vi "Teleop.vi"(10 "Match Info":T2={"Autonomous Elapsed Seconds"=0.0, "TeleOp Elapsed Seconds"=0.0, "Disabled Elapsed Seconds"=0.0, "Visited Autonomous"=FALSE, "Visited TeleOp"=FALSE, "Visited Disabled"=FALSE, "Autonomous Settings"={"Autonomous Style"=enum."Independent", "VI Refnum"=refnum}}, 11 "Call Context":T3) -> ()   [LabVIEW 2020]
doc: "This VI is called for each TeleOp packet received from the DS where the robot is not disabled. It is often used to read from the joysticks and update I/O or to update setpoints for timed control loops. It should complete and return within 20 milliseconds or it may miss DS packets."
uses:
  <vilib>/Rock Robotics/Network Tables/NT Write Numeric Array.vi
  <vilib>/Rock Robotics/Network Tables/NT Write Boolean Array.vi
  <vilib>/Rock Robotics/Network Tables/NT Read Boolean.vi
  <vilib>/Rock Robotics/WPI/ThirdParty/Phoenix-LabVIEW/Motor Controller/Controls/CTRE_Phoenix_MotorControl_ControlMode.ctl
  <vilib>/Rock Robotics/WPI/RobotDrive/WPI_RobotDriveMecanumDrive_Cartesian.vi
  <vilib>/Rock Robotics/Network Tables/NT Read Number.vi
  <vilib>/Rock Robotics/WPI/Solenoid/WPI_SolenoidSetEnum.vi
  <vilib>/Rock Robotics/WPI/DriverStation/WPI_DriverStationMatch Info.ctl
  <vilib>/Rock Robotics/WPI/DriverStation/WPI_DriverStationDerivedRobotMode.ctl
  <vilib>/Rock Robotics/WPI/Solenoid/WPI_SolenoidValue.ctl
panel:
  out "Distance 2":dbl
  out "Distance":dbl
  out "Angle":dbl=360.0
  in  "Camera servo up":i32
  out "Index Reverse":bool
  out "Index Foward":bool
  in  "Indexer Reverse":i32=6
  in  "Indexer forward":i32=4
  out "climb_cylinder":T1
  out "intake_cylinder":T1
  out "Indexer":dbl
  out "intake_motor_output":dbl
  out "Sample Slider 0":dbl(slide) scale=0.0..5.0
  out "Sample Boolean 1":bool
  out "Sample Boolean 0":bool
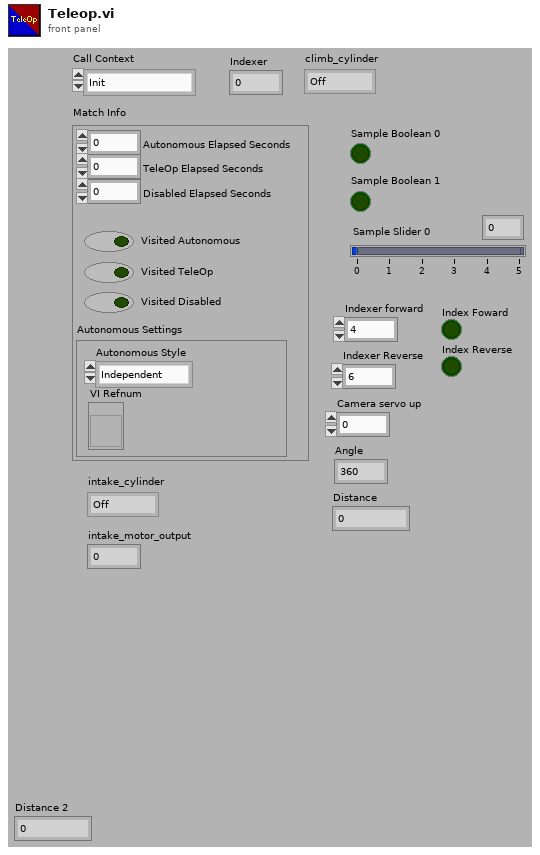
[diagram p1: front panel]
types:
  T1 = typedef "WPI_SolenoidValue.ctl" = enum16{"Off", "On", "Forward", "Reverse"}
  T2 = typedef "WPI_DriverStationMatch Info.ctl" = cluster{"Autonomous Elapsed Seconds":dbl, "TeleOp Elapsed Seconds":dbl, "Disabled Elapsed Seconds":dbl, "Visited Autonomous":bool, "Visited TeleOp":bool, "Visited Disabled":bool, "Autonomous Settings":cluster{"Autonomous Style":enum16{"Iterative", "Independent"}, "VI Refnum":refnum<vi>}}
  T3 = typedef "WPI_DriverStationDerivedRobotMode.ctl" = enum16{"Init", "Execute", "Stop"}
  T4 = typedef "CTRE_Phoenix_MotorControl_ControlMode.ctl" = u16
  T5 = typedef "WPI_GyroDevRef.ctl" = cluster{"DevStatus":errorcluster, "Analog Channel":T6, "Gain (VoltsPerDegree/Second)":dbl, "Gyro Type":enum16{"Analog", "XRS450"}, "Handle":i32, "SPI Bus":T7, "Device Found":bool, "Sample Rate":dbl, "Calibrate On Open":bool, "Offset":dbl}
  T6 = typedef "FPGA_AIChannel.ctl" = enum8{"AI 0", "AI 1", "AI 2", "AI 3", "AI MXP 0", "AI MXP 1", "AI MXP 2", "AI MXP 3", "Invalid"}
  T7 = typedef "spi_bus.ctl" = enum16{"SPI On-Board, CS0", "SPI On-Board, CS1", "SPI On-Board, CS2", "SPI On-Board, CS3", "SPI MXP", "Invalid"}
  T8 = typedef "WPI_EncoderDevRef.ctl" = cluster{"DevStatus":errorcluster, "EncoderIndex":T9, "CounterIndex":T10, "DistancePerCount":dbl, "Decoding Type":T11}
  T9 = typedef "FPGA_EncoderIdx.ctl" = enum8{"Enc 0", "Enc 1", "Enc 2", "Enc 3", "Enc 4", "Enc 5", "Enc 6", "Enc 7", "Invalid"}
  T10 = typedef "FPGA_CounterCtrSystemIndex.ctl" = enum8{"Ctr 0", "Ctr 1", "Ctr 2", "Ctr 3", "Ctr 4", "Ctr 5", "Ctr 6", "Ctr 7", "Invalid"}
  T11 = typedef "WPI_EncoderType.ctl" = enum16{"1x", "2x", "4x"}
  T12 = typedef "WPI_RobotDriveDevRef.ctl" = cluster{"DevStatus":errorcluster, "Motors[]":T13[], "Square Inputs":bool, "Max Output":dbl}
  T13 = typedef "WPI_MotorControlDeviceRef.ctl" = cluster{"DeviceStatus":errorcluster, "Type":T14, "PWM":cluster{"PWM Channel":T15, "DeadBand":T16}, "CAN":cluster{"Device Number":u8, "SetOutput VI Ref":variant, "GetOutput VI Ref":variant, "Enable VI Ref":variant, "Disable VI Ref":variant, "Data":variant}, "Invert":bool, "DIO PWM":cluster{"PWM \"Enable\" Channel":T15, "DIOChannel":T17, "PWM Rate":dbl}}
  T14 = typedef "WPI_MotorControlType.ctl" = enum16{"PWM", "CAN", "DIO PWM"}
  T15 = typedef "FPGA_DIOPWMChannel.ctl" = enum8{"PWM 0", "PWM 1", "PWM 2", "PWM 3", "PWM 4", "PWM 5", "PWM 6", "PWM 7", "PWM 8", "PWM 9", "PWM MXP 0", "PWM MXP 1", "PWM MXP 2", "PWM MXP 3", "PWM MXP 4", "PWM MXP 5", "PWM MXP 6", "PWM MXP 7", "PWM MXP 8", "PWM MXP 9", "Invalid"}
  T16 = typedef "WPI_PWMDeadband.ctl" = cluster{"Name":string, "maxPositivePwm":i32, "minPositivePwm":i32, "centerPwm":i32, "maxNegativePwm":i32, "minNegativePwm":i32, "angularRange":u16}
  T17 = typedef "FPGA_DIOChannel.ctl" = enum8{"DIO 0", "DIO 1", "DIO 2", "DIO 3", "DIO 4", "DIO 5", "DIO 6", "DIO 7", "DIO 8", "DIO 9", "DIO MXP 0", "DIO MXP 1", "DIO MXP 2", "DIO MXP 3", "DIO MXP 4", "DIO MXP 5", "DIO MXP 6", "DIO MXP 7", "DIO MXP 8", "DIO MXP 9", "DIO MXP 10", "DIO MXP 11", "DIO MXP 12", "DIO MXP 13", "DIO MXP 14", "DIO MXP 15", "SPI Port CS1", "SPI Port CS2", "SPI Port CS3", "SPI Port MISO", "SPI Port MOSI", "Invalid"}
  T18 = typedef "WPI_JoystickDevRef.ctl" = cluster{"Device":T19}
  T19 = typedef "WPI_JoystickDeviceEnum.ctl" = enum16{"USB 0", "USB 1", "USB 2", "USB 3", "USB 4", "USB 5"}
  T20 = typedef "WPI_ServoDeviceRef.ctl" = cluster{"DeviceStatus":errorcluster, "PWM Channel":T15, "DeadBand":T16}
  T21 = typedef "WPI_SolenoidDevRef.ctl" = cluster{"DevStatus":errorcluster, "Pneumatics Control Module":u8, "Forward Solenoid Channel":T22, "Reverse Solenoid Channel":T22}
  T22 = typedef "WPI_SolenoidChannel.ctl" = enum8{"Solenoid 0", "Solenoid 1", "Solenoid 2", "Solenoid 3", "Solenoid 4", "Solenoid 5", "Solenoid 6", "Solenoid 7", "Solenoid 8", "Solenoid 9", "Solenoid 10", "Solenoid 11", "Solenoid 12", "Solenoid 13", "Solenoid 14", "Solenoid 15", "Invalid"}
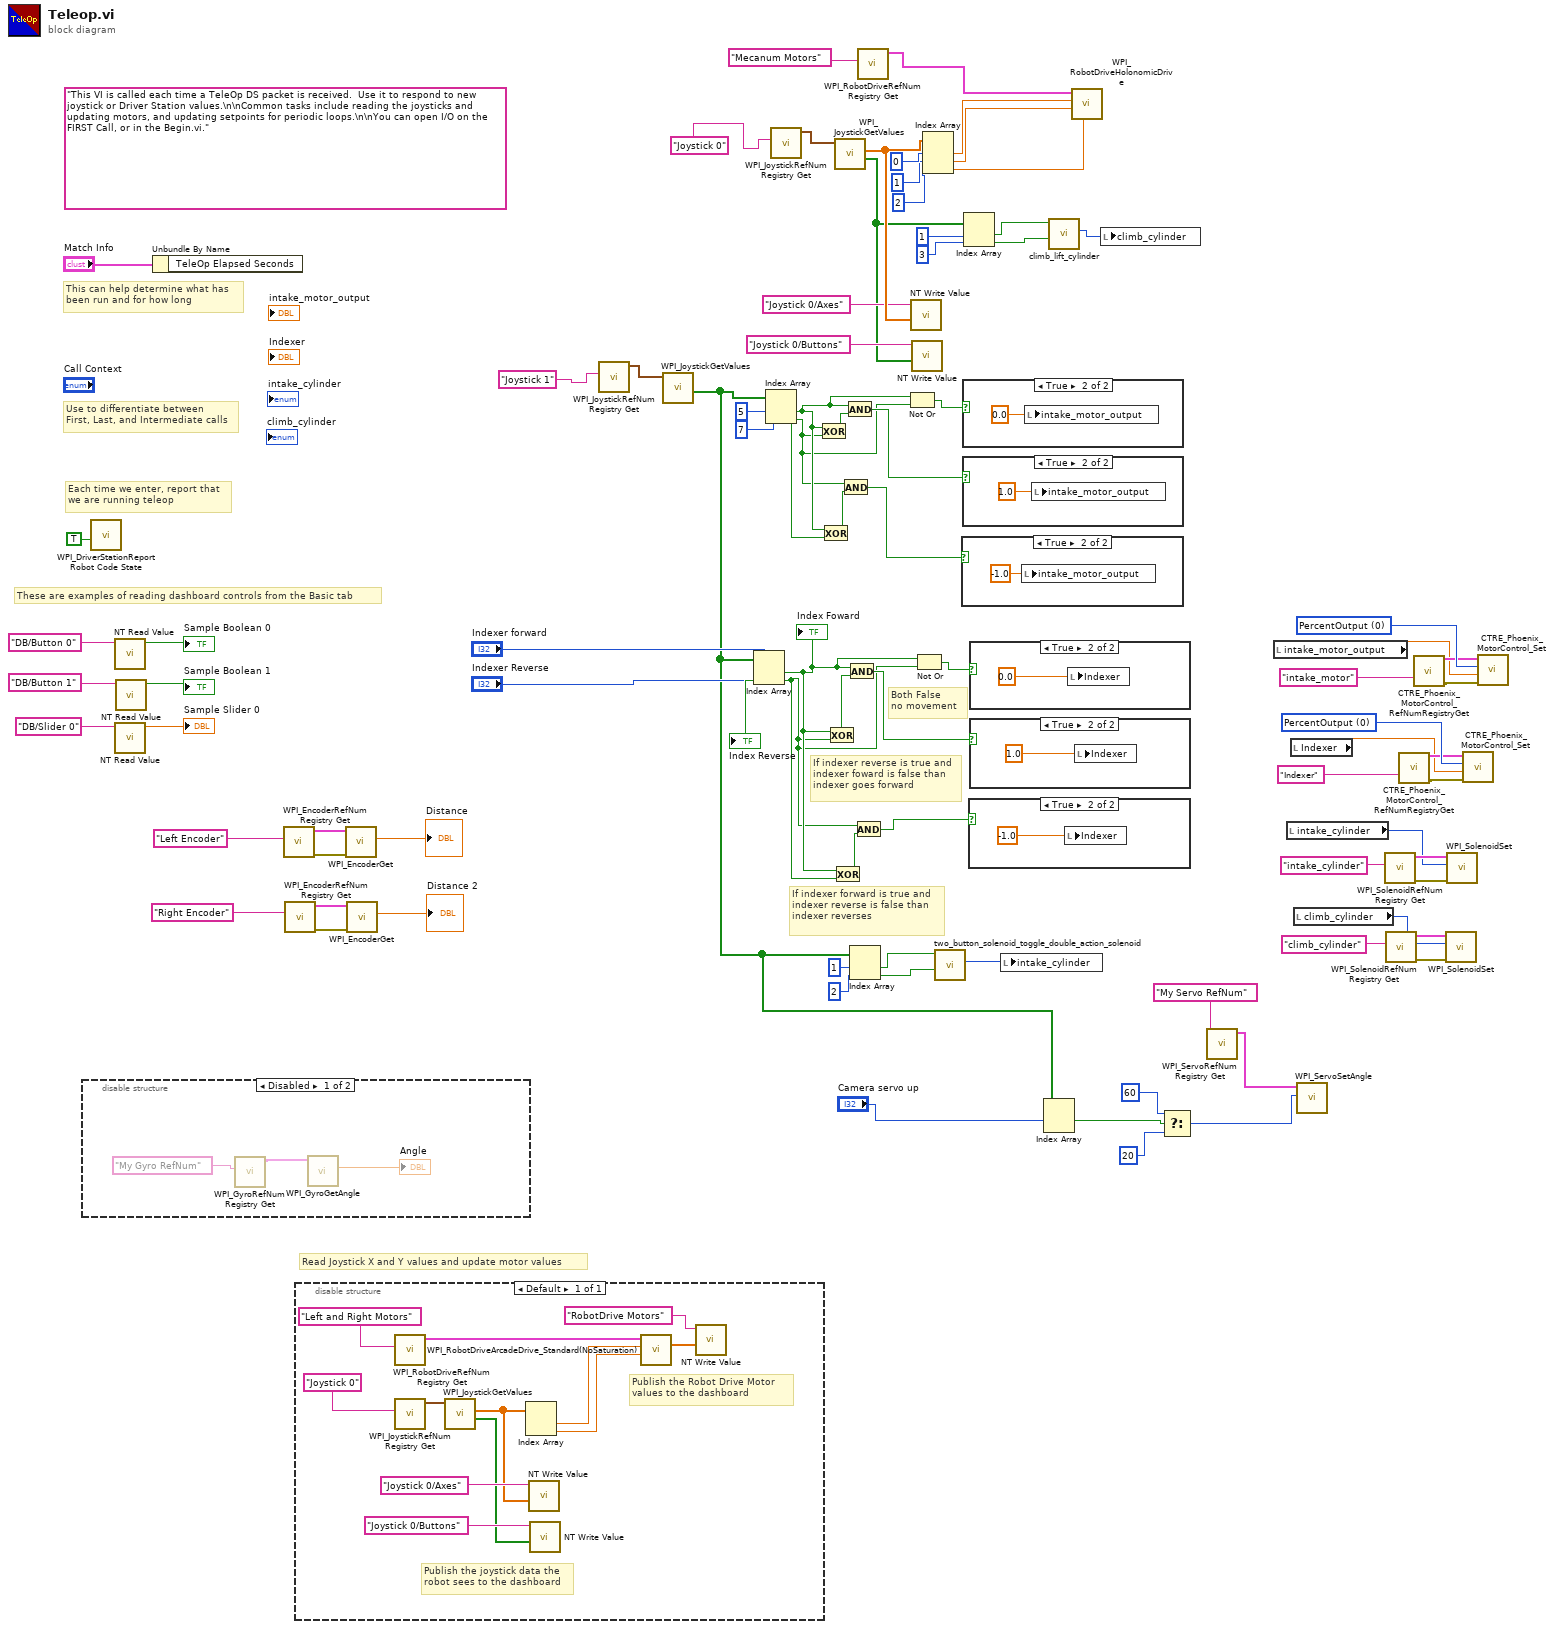
[diagram p0: block diagram]
diagram:
  w49 = T4 0 items=["PercentOutput"=0, "Position"=1, "Velocity"=2, "Current"=3, "Follower"=5, "MotionProfile"=6, "MotionMagic"=7, "MotionProfileArc"=10, "Disabled"=15] ("Control Mode")
  w58 = T4 0 items=["PercentOutput"=0, "Position"=1, "Velocity"=2, "Current"=3, "Follower"=5, "MotionProfile"=6, "MotionMagic"=7, "MotionProfileArc"=10, "Disabled"=15] ("Control Mode")
  (unwired) "This VI is called each time a TeleOp DS packet is received.  Use it to respond to new joystick or Driver Station values.\n\nCommon tasks include reading the joysticks and updating motors, and updating setpoints for periodic loops.\n\nYou can open I/O on the FIRST Call, or in the Begin.vi."
  # "If indexer reverse is true and\nindexer foward is false than \nindexer goes forward"
  # "Both False\nno movement"
  # "If indexer forward is true and\nindexer reverse is false than \nindexer reverses"
  # "These are examples of reading dashboard controls from the Basic tab"
  # "Each time we enter, report that\nwe are running teleop"
  # "Use to differentiate between\nFirst, Last, and Intermediate calls"
  # "This can help determine what has\nbeen run and for how long"
  # "Read Joystick X and Y values and update motor values"
  n1 = disable-structure shown="Disabled" {
    frame Disabled {
      n2 = call <vilib>:"WPI_GyroRefNum Registry Get.vi"("refnum name"="My Gyro RefNum") -> ("GyroDevRef"=w88:T5)  [unwired: 9 in, 1 out]
      n3 = call <vilib>:"WPI_GyroGetAngle.vi"("GyroDevRef"=w88) -> ("Angle"=→"Angle":dbl)  [unwired: 6 in, 4 out]
    }
    frame Enabled {
    }
  }
  n4 = call <vilib>:"WPI_DriverStationReport Robot Code State.vi"("TeleOp"=TRUE ("Autonomous")) -> ()  [unwired: 10 in, 1 out]
  n5 = call-poly <vilib>:"NT Read Value.vi"("name"="DB/Button 0" ("refnum name")) -> ("value"=→"Sample Boolean 0":bool)  [unwired: 8 in, 2 out]
  n6 = call-poly <vilib>:"NT Read Value.vi"("name"="DB/Slider 0" ("refnum name")) -> ("value"=→"Sample Slider 0":dbl)  [unwired: 8 in, 2 out]
  n7 = call-poly <vilib>:"NT Read Value.vi"("name"="DB/Button 1" ("refnum name")) -> ("value"=→"Sample Boolean 1":bool)  [unwired: 8 in, 2 out]
  n8 = Unbundle By Name("Match Info") -> ()  [unwired: 1 out]
  n9 = call <vilib>:"WPI_EncoderRefNum Registry Get.vi"("refnum name"="Left Encoder") -> ("error out"=w6:errorcluster, "EncoderDevRef"=w7:T8)  [unwired: 9 in]
  n10 = call <vilib>:"WPI_EncoderRefNum Registry Get.vi"("refnum name"="Right Encoder") -> ("error out"=w3:errorcluster, "EncoderDevRef"=w4:T8)  [unwired: 9 in]
  n11 = disable-structure shown="Default" {
    frame Enabled {
      # "Publish the Robot Drive Motor\nvalues to the dashboard"
      # "Publish the joystick data the\nrobot sees to the dashboard"
      n12 = call <vilib>:"WPI_RobotDriveRefNum Registry Get.vi"("refnum name"="Left and Right Motors") -> ("RobotDriveDevRef"=w100:T12)  [unwired: 1 in, 9 out]
      n13 = call <vilib>:"WPI_JoystickRefNum Registry Get.vi"("refnum name"="Joystick 0") -> ("JoystickDevRef"=w97:T18)  [unwired: 1 in, 9 out]
      n14 = call <vilib>:"WPI_JoystickGetValues.vi"("JoystickDevRef"=w97) -> ("Buttons"=w92:bool[], "Axes"=w93:dbl[])  [unwired: 6 in, 3 out]
      n15 = Index Array(array=w93) -> (element #1=w99:dbl, element #2=w96:dbl)  [unwired: 2 in]
      n16 = call-poly <vilib>:"NT Write Value.vi"("value"=w93, "name"="Joystick 0/Axes" ("Name")) -> ()  [unwired: 9 in, 1 out]
      n17 = call-poly <vilib>:"NT Write Value.vi"("value"=w92, "name"="Joystick 0/Buttons" ("Name")) -> ()  [unwired: 9 in, 1 out]
      n18 = call <vilib>:"WPI_RobotDriveArcadeDrive_Standard(NoSaturation).vi"("Y axis value"=w96, "X axis value"=w99, "RobotDriveDevRef"=w100) -> ("Motor Values"=w91:dbl[])  [unwired: 1 in, 7 out]
      n19 = call-poly <vilib>:"NT Write Value.vi"("value"=w91, "name"="RobotDrive Motors" ("Name")) -> ()  [unwired: 9 in, 1 out]
    }
  }
  n20 = call <vilib>:"WPI_EncoderGet.vi"("error in (no error)"=w6, "EncoderDevRef"=w7) -> ("Distance"=→"Distance":dbl)  [unwired: 4 in, 5 out]
  n21 = call <vilib>:"WPI_EncoderGet.vi"("error in (no error)"=w3, "EncoderDevRef"=w4) -> ("Distance"=→"Distance 2":dbl)  [unwired: 4 in, 5 out]
  n22 = call <vilib>:"WPI_JoystickRefNum Registry Get.vi"("refnum name"="Joystick 1") -> ("JoystickDevRef"=w54:T18)  [unwired: 1 in, 9 out]
  n23 = call <vilib>:"WPI_JoystickGetValues.vi"("JoystickDevRef"=w54) -> ("Buttons"=w13:bool[])  [unwired: 6 in, 4 out]
  n24 = Index Array(array=w13, index #1="Indexer forward", index #2="Indexer Reverse") -> (element #1=w40:bool, element #2=w39:bool)
  "Index Foward" <- w40
  "Index Reverse" <- w39
  n25 = Index Array(array=w13, index #1=5 ("index"), index #2=7 ("index")) -> (element #1=w61:bool, element #2=w60:bool)
  n26 = call <vilib>:"WPI_JoystickRefNum Registry Get.vi"("refnum name"="Joystick 0") -> ("JoystickDevRef"=w75:T18)  [unwired: 1 in, 9 out]
  n27 = Exclusive Or(1:w60, 2:w61) -> (0:w65:bool)
  n28 = Exclusive Or(1:w60, 2:w61) -> (0:w64:bool)
  n29 = Exclusive Or(1:w39, 2:w40) -> (0:w44:bool)
  n30 = Exclusive Or(1:w39, 2:w40) -> (0:w43:bool)
  n31 = call <vilib>:"WPI_JoystickGetValues.vi"("JoystickDevRef"=w75) -> ("Buttons"=w23:bool[], "Axes"=w71:dbl[])  [unwired: 6 in, 3 out]
  n32 = And(x=w60, y=w64) -> (x .and. y?=w62:bool)
  n33 = And(x=w61, y=w65) -> (x .and. y?=w63:bool)
  n34 = And(x=w40, y=w44) -> (x .and. y?=w42:bool)
  n35 = Index Array(array=w13, index #1=1 ("index"), index #2=2 ("index")) -> (element #1=w35:bool, element #2=w34:bool)
  n36 = And(x=w39, y=w43) -> (x .and. y?=w41:bool)
  n37 = call <vilib>:"WPI_RobotDriveRefNum Registry Get.vi"("refnum name"="Mecanum Motors") -> ("RobotDriveDevRef"=w73:T12)  [unwired: 1 in, 9 out]
  n38 = Not Or(1:w60, 2:w61) -> (0:w59:bool)
  n39 = call-poly <vilib>:"NT Write Value.vi"("value"=w71, "name"="Joystick 0/Axes" ("Name")) -> ()  [unwired: 9 in, 1 out]
  n40 = call-poly <vilib>:"NT Write Value.vi"("value"=w23, "name"="Joystick 0/Buttons" ("Name")) -> ()  [unwired: 9 in, 1 out]
  n41 = Not Or(1:w39, 2:w40) -> (0:w38:bool)
  n42 = Index Array(array=w71, index #1=0 ("index"), index #2=1 ("index"), index #3=2 ("index")) -> (element #1=w78:dbl, element #2=w77:dbl, element #3=w76:dbl)
  n43 = call "two_button_solenoid_toggle_double_action_solenoid.vi"("Button A"=w35, "Button B"=w34) -> ("Cylinder_out"=w37:T1)  [unwired: 8 in]
  n44 = case shown="True" w62 {
    frame False {
    }
    frame True {
      n45 = local write "intake_motor_output"(-1.0) -> ()
    }
  }
  n46 = case shown="True" w59 {
    frame False {
    }
    frame True {
      n47 = local write "intake_motor_output"(0.0) -> ()
    }
  }
  n48 = case shown="True" w63 {
    frame False {
    }
    frame True {
      n49 = local write "intake_motor_output"(1.0) -> ()
    }
  }
  n50 = Index Array(array=w23, index #1=1 ("index"), index #2=3 ("index")) -> (element #1=w28:bool, element #2=w27:bool)
  n51 = case shown="True" w41 {
    frame False {
    }
    frame True {
      n52 = local write "Indexer"(-1.0) -> ()
    }
  }
  n53 = case shown="True" w38 {
    frame False {
    }
    frame True {
      n54 = local write "Indexer"(0.0) -> ()
    }
  }
  n55 = case shown="True" w42 {
    frame False {
    }
    frame True {
      n56 = local write "Indexer"(1.0) -> ()
    }
  }
  n57 = local write "intake_cylinder"(w37) -> ()
  n58 = Index Array(array=w13, index #1="Camera servo up") -> (element #1=w11:bool)  [unwired: 1 in, 1 out]
  n59 = call "climb_lift_cylinder.vi"("Button A"=w28, "Button B"=w27) -> ("climb_lyft_cylinder"=w24:T1)  [unwired: 8 in]
  n60 = call-poly <vilib>:"WPI_RobotDriveHolonomicDrive.vi"("Rotation"=w76, "Y"=w77, "X"=w78, "RobotDriveDevRef"=w73) -> ()  [unwired: 5 in, 3 out]
  n61 = local write "climb_cylinder"(w24) -> ()
  n62 = Select(t=60, s=w11, f=20) -> (s? t:f=w10:i32)
  n63 = call <vilib>:"WPI_ServoRefNum Registry Get.vi"("refnum name"="My Servo RefNum") -> ("ServoDeviceRef"=w14:T20)  [unwired: 9 in, 1 out]
  n64 = local read "intake_motor_output"() -> (w55:dbl)
  n65 = local read "intake_cylinder"() -> (w31:T1)
  n66 = local read "Indexer"() -> (w46:dbl)
  n67 = local read "climb_cylinder"() -> (w21:T1)
  n68 = call <vilib>:"WPI_ServoSetAngle.vi"("Angle"=w10, "ServoDeviceRef"=w14) -> ()  [unwired: 8 in, 2 out]
  n69 = call <vilib>:"WPI_SolenoidRefNum Registry Get.vi"("refnum name"="intake_cylinder") -> ("error out"=w33:errorcluster, "SolenoidDevRef"=w32:T21)  [unwired: 9 in]
  n70 = call <vilib>:"WPI_SolenoidRefNum Registry Get.vi"("refnum name"="climb_cylinder") -> ("error out"=w19:errorcluster, "SolenoidDevRef"=w22:T21)  [unwired: 9 in]
  n71 = call <vilib>:"CTRE_Phoenix_MotorControl_RefNumRegistryGet.vi"("refnum name"="Indexer") -> ("error out"=w47:errorcluster, "PhoenixMotorControlDevRef"=w48:T13)  [unwired: 9 in]
  n72 = call <vilib>:"CTRE_Phoenix_MotorControl_RefNumRegistryGet.vi"("refnum name"="intake_motor") -> ("error out"=w56:errorcluster, "PhoenixMotorControlDevRef"=w57:T13)  [unwired: 9 in]
  n73 = call-poly <vilib>:"WPI_SolenoidSet.vi"("error in (no error)"=w19, "Value"=w21, "SolenoidDevRef"=w22) -> ()  [unwired: 7 in, 2 out]
  n74 = call-poly <vilib>:"WPI_SolenoidSet.vi"("error in (no error)"=w33, "Value"=w31, "SolenoidDevRef"=w32) -> ()  [unwired: 7 in, 2 out]
  n75 = call <vilib>:"CTRE_Phoenix_MotorControl_Set.vi"("error in (no error)"=w47, "Output"=w46, "Control Mode"=w49, "PhoenixMotorControlDevRef"=w48) -> ()  [unwired: 6 in, 2 out]
  n76 = call <vilib>:"CTRE_Phoenix_MotorControl_Set.vi"("error in (no error)"=w56, "Output"=w55, "Control Mode"=w58, "PhoenixMotorControlDevRef"=w57) -> ()  [unwired: 6 in, 2 out]
